vi "Timer test.vi"() -> ()   [LabVIEW 2024]
panel:
  in  "stop":bool
  in  "reset button":bool
  out "Indicator":dbl
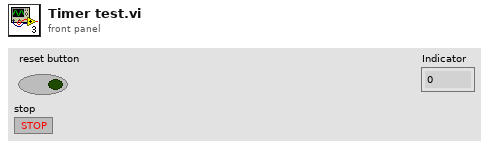
[diagram p1: front panel]
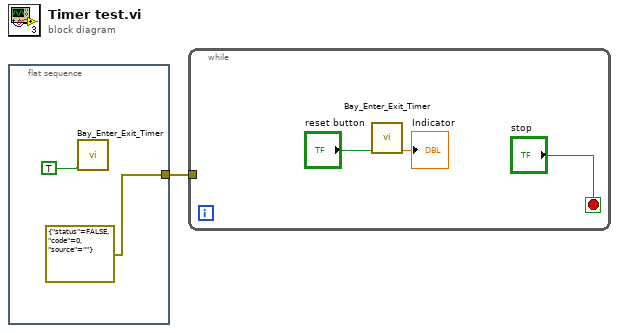
[diagram p0: block diagram]
diagram:
  n1 = flat-sequence {
    tunnel: [errorcluster {"status"=FALSE, "code"=0, "source"=""} ("error constant")] -> w1
    frame #0 {
      n2 = call "Bay_Enter_Exit_Timer.vi"("reset button"=TRUE) -> ()  [unwired: 10 in, 1 out]
    }
  }
  n3 = while {
    tunnel: w1 -> [_]
    stop <- "stop" stop-if-true
    n4 = call "Bay_Enter_Exit_Timer.vi"("reset button"="reset button") -> ("Indicator"=→"Indicator":dbl)  [unwired: 10 in]
  }
